vi "灯值调整对话框.vi"() -> ()   [LabVIEW 2016, in "斯坦道总氮.lvlib"]
panel:
  out "660 阻值":u16 caption="660 阻值："
  out "520 阻值":u16 caption="520 阻值："
  out "360 阻值":u16 caption="360 阻值："
  in  "停止":bool
  in  "校准":bool
  out "校准状态":u16(ring) caption="当前状态：" items=["空闲", "校准中"]
  out "当前阻值":u16 caption="当前阻值："
  out "当前光强":u16 caption="当前光强："
  in  "目标光强":u16 caption="目标光强："
  in  "灯类型":enum32{"360", "520", "660"}(radio) caption="灯类型："
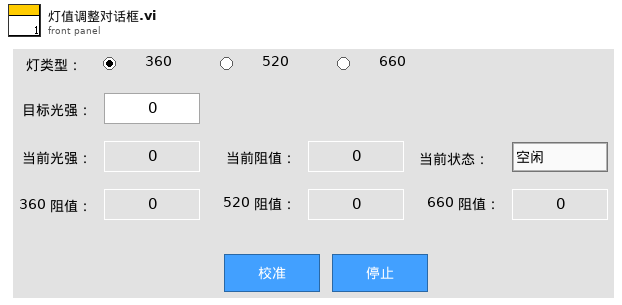
[diagram p1: front panel]
types:
  T1 = cluster{"360 阻值":u16, "520 阻值":u16, "660 阻值":u16}
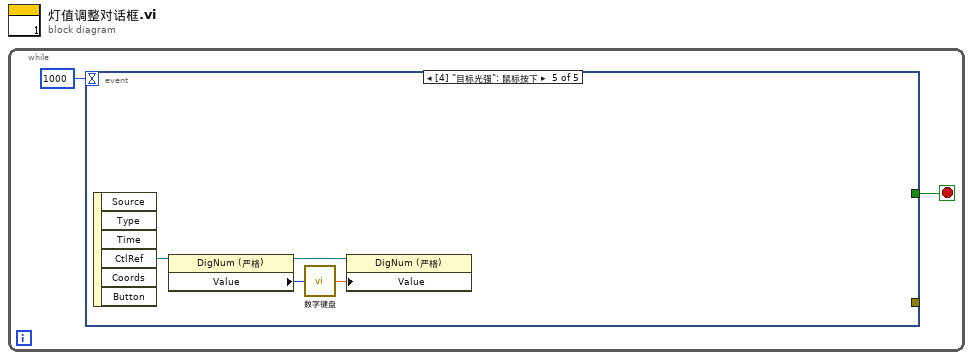
[diagram p0: block diagram]
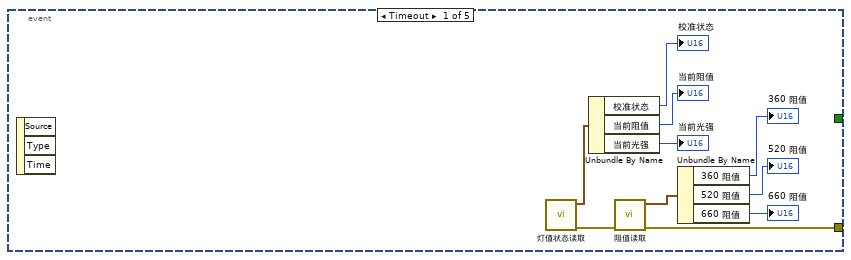
[diagram p2: hidden frame]
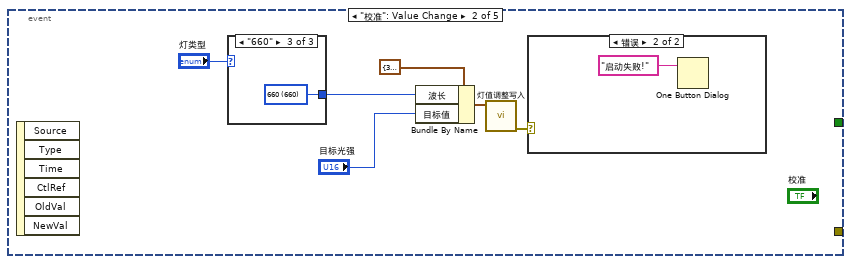
[diagram p3: hidden frame]
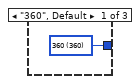
[diagram p5: hidden frame]
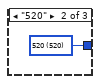
[diagram p6: hidden frame]
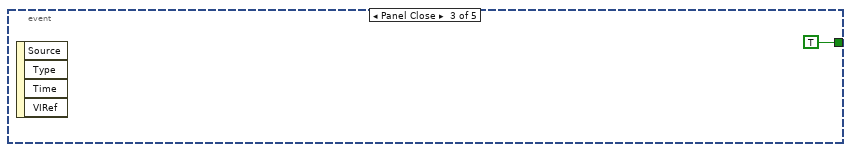
[diagram p7: hidden frame]
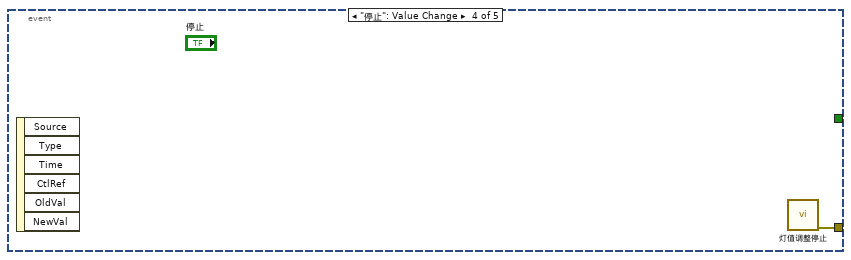
[diagram p8: hidden frame]
diagram:
  n1 = while {
    stop <- w2 stop-if-true
    n2 = event shown="[4] \"目标光强\": 鼠标按下" {
      selector: _ -> [_ _ _ _ _]
      dyn-events: _ -> [_ _ _ _ _]
      timeout: 1000 -> [_ _ _ _ _]
      tunnel: [_ _ TRUE _ _] -> w2
      tunnel: [w3 _ _ w24 _] -> _
      event Timeout {
        n3 = event-data() -> ()  [unwired: 1 in, 3 out]
        n4 = call "灯值状态读取.vi"() -> ("error out"=w12:errorcluster, "状态值"=w11:cluster{"校准状态":u16, "当前阻值":u16, "当前光强":u16})  [unwired: 10 in]
        n5 = Unbundle By Name(w11) -> ("校准状态"=→"校准状态":u16, "当前阻值"=→"当前阻值":u16, "当前光强"=→"当前光强":u16)
        n6 = call "阻值读取.vi"("error in (no error)"=w12) -> ("error out"=w3:errorcluster, "状态值"=w7:T1)  [unwired: 9 in]
        n7 = Unbundle By Name(w7) -> ("360 阻值"=→"360 阻值":u16, "520 阻值"=→"520 阻值":u16, "660 阻值"=→"660 阻值":u16)
      }
      event "校准": Value Change {
        n8 = event-data() -> ()  [unwired: 1 in, 6 out]
        n9 = case shown="\"660\"" "灯类型" {
          tunnel: [w20 w21 w22] -> w16
          frame "360", Default {
            w20 = u16 360 items=["360"=360, "520"=520, "660"=660] ("波长")
          }
          frame "520" {
            w21 = u16 520 items=["360"=360, "520"=520, "660"=660] ("波长")
          }
          frame "660" {
            w22 = u16 660 items=["360"=360, "520"=520, "660"=660] ("波长")
          }
        }
        n10 = Bundle By Name(cluster=cluster{"波长":u16, "ADC":u16, "目标值":u16} {"波长"=360, "ADC"=0, "目标值"=0} ("写入值"), "波长"=w16, "目标值"="目标光强") -> (w15:cluster{"波长":u16, "ADC":u16, "目标值":u16})
        n11 = call "灯值调整写入.vi"("写入值"=w15) -> ("error out"=w13:errorcluster)  [unwired: 10 in]
        n12 = case shown="错误" w13 {
          frame No Error {
          }
          frame Error {
            n13 = One Button Dialog(message="启动失败!" ("消息")) -> ()  [unwired: 1 in, 1 out]
          }
        }
      }
      event Panel Close {
        n14 = event-data() -> ()  [unwired: 1 in, 4 out]
      }
      event "停止": Value Change {
        n15 = event-data() -> ()  [unwired: 1 in, 6 out]
        n16 = call "灯值调整停止.vi"() -> ("error out"=w24:errorcluster)  [unwired: 11 in]
      }
      event "目标光强": Mouse Down {
        n17 = event-data() -> ("CtlRef"=w28:refnum<vi>)  [unwired: 1 in, 5 out]
        n18 = property class="DigNum (严格)"(reference=w28) -> (reference out=w25:refnum<vi>, "Value"=w27:u16)  [unwired: 1 in, 1 out]
        n19 = call "数字键盘.vi"("OldNumber"=w27) -> ("NewNumber"=w26:dbl)
        n20 = property class="DigNum (严格)"(reference=w25, "Value"=w26) -> ()  [unwired: 1 in, 2 out]
      }
    }
  }
